vi "BASE.Create.vi"(8 "error in (no error)":errorcluster, 11 "BASE.Device in":refnum<class "BASE.Device.lvclass">) -> (0 "error out":errorcluster, 3 "BASE.Device out":refnum<class "BASE.Device.lvclass">)   [LabVIEW 2019, in "BASE.Device.lvlib" / "BASE.Device.lvclass"]
uses:
  BASE.Device.lvclass
  BASE.Device.lvclass/BASE.Device.ctl
  BASE/BASE/BASE.lvclass
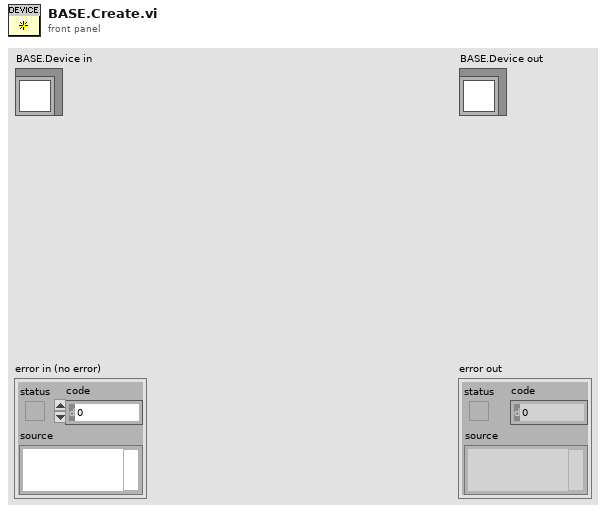
[diagram p1: front panel]
types:
  T1 = typedef "BASE.Device.lvlib/BASE.Device.lvclass/privateData--reference.ctl" = refnum<data-value>
  T2 = typedef "BASE.Device.lvlib/BASE.Device.lvclass/privateData--cluster.ctl" = cluster{"config":T3, "Connected?":bool}
  T3 = typedef "BASE.Device.lvlib/BASE.Device.lvclass/config--cluster.ctl" = cluster{"Connect Timeout":i32, "Connect Interval":u32, "Check Timeout":i32, "Check Intverval":u32, "Read Timeout":i32, "Read Interval":u32}
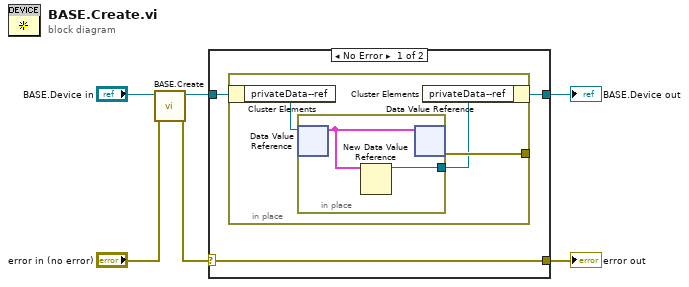
[diagram p0: block diagram]
diagram:
  n1 = call-parent "BASE.Create.vi"("error in (no error)"="error in (no error)", "BASE in"="BASE.Device in") -> ("error out"=w4:errorcluster, "BASE out"=w3:refnum<class "BASE.Device.lvclass">)  [unwired: 8 in]
  n2 = case shown="No Error" w4 {
    selector: w4 -> [w7 w15]
    tunnel: w3 -> [w9 w16]
    tunnel: [w8 w16] -> w2
    tunnel: [w7 w15] -> w1
    frame No Error {
      n3 = in-place {
        in-place-border: [w11] -> _
        n4 = in-place-cluster #1(w9) -> ("privateData--ref"=w12:T1)
        n5 = in-place {
          in-place-border: [w14] -> w10
          n6 = in-place-dvr #2(w12) -> (w13:T2)  [unwired: 1 out]
          n7 = New Data Value Reference(data value=w13) -> (data value reference=w14:refnum<data-value>)  [unwired: 1 in, 1 out]
          n8 = in-place-dvr #2(w13) -> (w11:errorcluster)  [unwired: 1 out]
        }
        n9 = in-place-cluster #1("privateData--ref"=w10) -> (w8:refnum<class "BASE.Device.lvclass">)
      }
    }
    frame Error {
    }
  }
  "error out" <- w1
  "BASE.Device out" <- w2
